vi "Configure.vi"(8 "error in (no error)":errorcluster, 10 "Params":variant, 11 "DAQmx Base in":refnum<class "DAQmx Base.lvclass">) -> (0 "error out":errorcluster, 3 "DAQmx Base out":refnum<class "DAQmx Base.lvclass">)   [LabVIEW 2020]
uses:
  DAQmx Base.lvclass
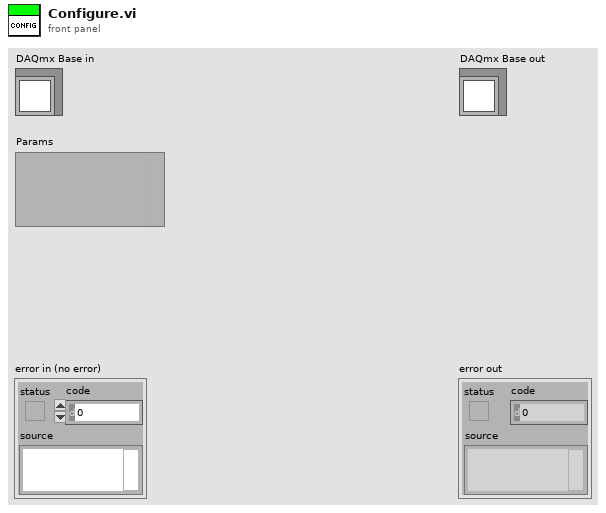
[diagram p1: front panel]
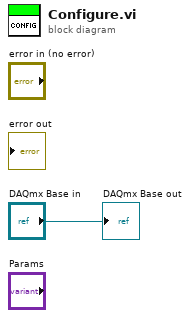
[diagram p0: block diagram]
diagram:
  "DAQmx Base out" <- "DAQmx Base in"
